vi "Stop.vi"(8 "error in (no error)":errorcluster, 10 "Message in":refnum<class "StopMessage.lvclass">, 11 "StageSPIM in":refnum<class "StageSPIM.lvclass">) -> (0 "error out":errorcluster, 3 "StageSPIM out":refnum<class "StageSPIM.lvclass">)   [LabVIEW 2012, in "StageSPIM.lvclass"]
doc: "This member function is called when the statemachine in the run.vi receives an 'stop' command. It relays the message to all observers of the component.\n\nOverride this member function in your derived class if you need additional stop functionality (but don't forget to call the parent method)."
uses:
  StageSPIM.lvclass
  <vilib>/Distrio/Murmex/StopMessage/StopMessage.lvclass
  <vilib>/Distrio/Murmex/Murmex/Murmex.lvclass
  <vilib>/Distrio/Murmex/GenericMessage/GenericMessage.lvclass
  <vilib>/Distrio/Murmex/Message/Add or replace parameter.vi
panel:
  out "Controller error":bool
  # "This method is called when the STOP\ntrigger is sent. \n\nOverride this method when your component needs to\nrespond to this trigger. \n\nCall parent for proper implementation"
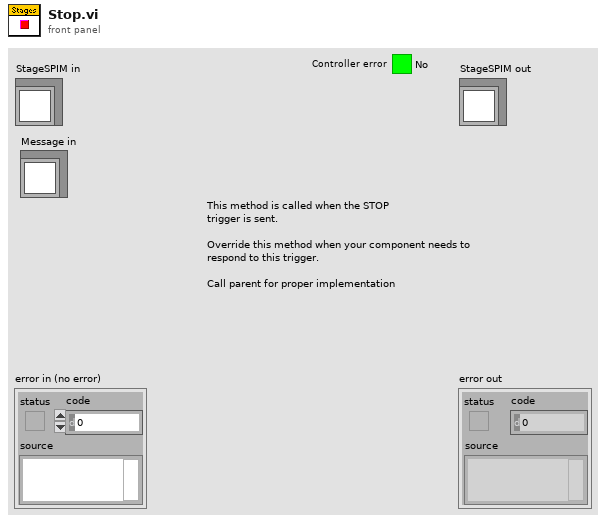
[diagram p1: front panel]
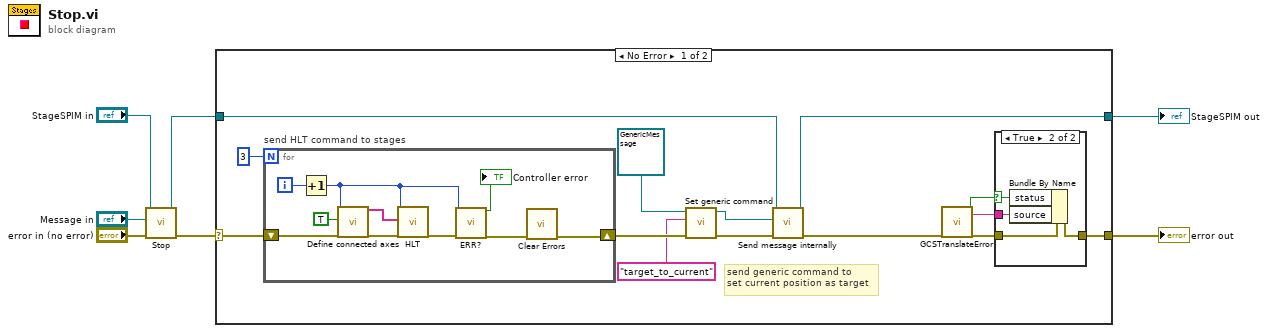
[diagram p0: block diagram]
diagram:
  n1 = call-parent "Stop.vi"("error in (no error)"="error in (no error)", "Message in"="Message in", "Murmex in"="StageSPIM in") -> ("error out"=w4:errorcluster, "Murmex out"=w3:refnum<class "StageSPIM.lvclass">)  [unwired: 7 in]
  n2 = case shown="No Error" w4 {
    selector: w4 -> [w21 w37]
    tunnel: w3 -> [w11 w38]
    tunnel: [w10 w38] -> w2
    tunnel: [w13 w37] -> w1
    frame No Error {
      # "send generic command to\nset current position as target"
      n3 = for "send HLT command to stages" {
        N: 3 -> [_]
        shift-right: [w27] -> w19
        shift-left: w21 -> [w34]
        i -> [w36]
        n4 = Increment(x=w36) -> (x+1=w30:i32)
        n5 = call "Define connected axes.vi"("System no."=w30, "Read from\ncontroller?"=TRUE ("Read from\ncontroller?"), "error in"=w34) -> ("Conn. Axes out"=w32:string[], "error out"=w35:errorcluster)  [unwired: 15 in]
        n6 = call "HLT.vi"("System no."=w30, "Affected axes"=w32, "error in"=w35) -> ("error out"=w31:errorcluster)  [unwired: 16 in]
        n7 = call "ERR?.vi"("System no."=w30, "error in"=w31) -> ("Controller error"=→"Controller error":bool, "error out"=w28:errorcluster)  [unwired: 16 in]
        n8 = call <vilib>:"Clear Errors.vi"("error in (no error)"=w28) -> ("error out"=w27:errorcluster)  [unwired: 6 in]
      }
      n9 = call <vilib>:"Set generic command.vi"("error in (no error)"=w19, "generic command"="target_to_current", "GenericMessage in"=refnum<class "GenericMessage.lvclass"> refnum ("Distrio Murmex 1.2:GenericMessage")) -> ("error out"=w12:errorcluster, "GenericMessage out"=w9:refnum<class "GenericMessage.lvclass">)  [unwired: 7 in]
      n10 = call <vilib>:"Send message internally.vi"("error in (no error)"=w12, "Message"=w9, "Murmex in"=w11) -> ("error out"=w8:errorcluster, "Murmex out"=w10:refnum<class "StageSPIM.lvclass">)  [unwired: 7 in]
      n11 = call "GCSTranslateError.vi"("error in"=w8) -> ("GCS Error?"=w15:bool, "Error Description"=w16:string, "error out"=w14:errorcluster)  [unwired: 16 in]
      n12 = case shown="True" w15 {
        selector: w15 -> [_ w24]
        tunnel: w14 -> [w22 w26]
        tunnel: [w22 w25] -> w13
        tunnel: w16 -> [_ w23]
        frame False {
        }
        frame True {
          n13 = Bundle By Name(cluster=w26, "status"=w24, "source"=w23) -> (w25:errorcluster)
        }
      }
    }
    frame Error {
    }
  }
  "error out" <- w1
  "StageSPIM out" <- w2
